vi "Set Line.vi"(8 "error in (no error)":errorcluster, 9 "Interlock Chain":refnum<class "Interlock Chain.lvclass">, 10 "Bit Field":u16, 11 "Storage Line in":refnum<class "Storage Line.lvclass">) -> (0 "error out":errorcluster, 3 "Storage Line out":refnum<class "Storage Line.lvclass">)   [LabVIEW 2015, in "cRIO-Carbondioxide.lvlib" / "CO2-Actor.lvlib" / "Storage Line.lvclass"]
uses:
  Storage Line.lvclass
  Interlocks/Interlock Chain/Interlock Chain.lvclass
  Storage Line.lvclass/Storage Line.ctl
  <vilib>/ActorFramework/Actor/Actor.lvclass/Actor.ctl
  <vilib>/ActorFramework/Message Enqueuer/Message Enqueuer.lvclass/Message Enqueuer.ctl
  Valve Messages/Write Bit Field Msg/Write Bit Field Msg.lvclass/Write Bit Field Msg.ctl
  <vilib>/ActorFramework/Actor/Read Self Enqueuer.vi
  <vilib>/ActorFramework/Message Enqueuer/Enqueue.vi
  Read Container.vi
  <vilib>/ActorFramework/Message Enqueuer/Init from Existing Queue.vi
  <vilib>/ActorFramework/Message Priority Queue/Priority Enqueue.vi
  Interlocks/Interlock/Interlock.lvclass
  <vilib>/ActorFramework/Actor/Actor.lvclass
  <vilib>/ActorFramework/Message Enqueuer/Message Enqueuer.lvclass
  Valve Messages/Write Bit Field Msg/Write Bit Field Msg.lvclass
  subs/Sample/Sample.lvclass
  CO2 Actor/CO2 Actor.lvclass
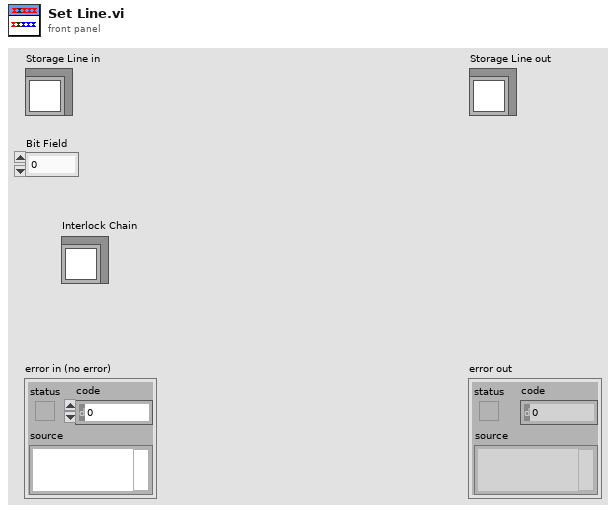
[diagram p1: front panel]
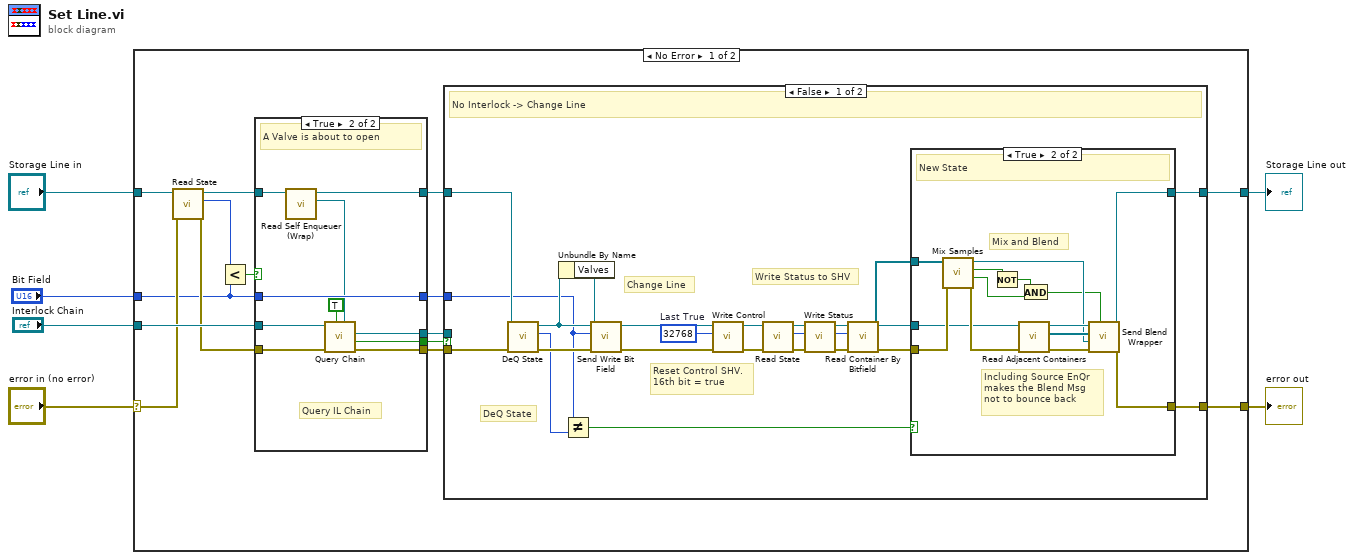
[diagram p0: block diagram]
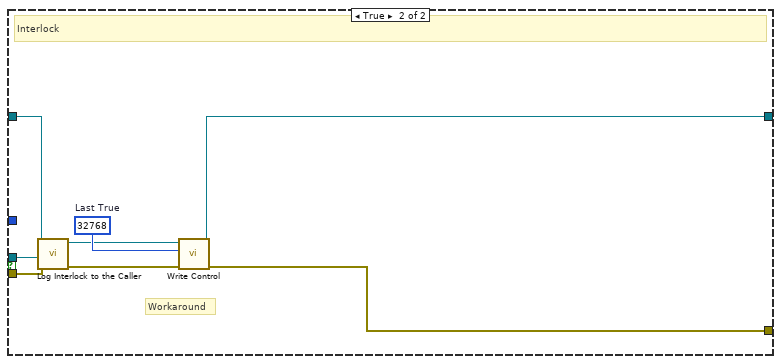
[diagram p4: hidden frame]
diagram:
  n1 = case shown="No Error" "error in (no error)" {
    selector: "error in (no error)" -> [w16 w83]
    tunnel: [w10 w83] -> w5
    tunnel: [w9 w82] -> w3
    tunnel: "Storage Line in" -> [w17 w82]
    tunnel: "Interlock Chain" -> [w21 _]
    tunnel: "Bit Field" -> [w13 _]
    frame No Error {
      n2 = call "Read State.vi"("error in (no error)"=w16, "Storage Line in"=w17) -> ("error out"=w15:errorcluster, "State"=w11:u16, "Storage Line out"=w8:refnum<class "Storage Line.lvclass">)  [unwired: 5 in, 2 out]
      n3 = Less?(x=w11, y=w13) -> (x < y?=w14:bool)
      n4 = case shown="True" w14 {
        tunnel: w21 -> [_ w34]
        tunnel: [w24 w32] -> w20
        tunnel: [_ w31] -> w19
        tunnel: [_ w30] -> w18
        tunnel: w15 -> [w24 w29]
        tunnel: w13 -> [w23 w28]
        tunnel: [w23 w28] -> w12
        tunnel: w8 -> [w22 w27]
        tunnel: [w22 w25] -> w7
        frame False {
          # "Nevermind Interlock"
          # "Valve is about to close"
        }
        frame True {
          # "Query IL Chain"
          # "A Valve is about to open"
          n5 = call "Read Self Enqueuer (Wrap).vi"("CO2 Actor in"=w27) -> ("Actor Framework:Message Enqueuer"=w26:refnum<class "Message Enqueuer.lvclass">, "CO2 Actor out"=w25:refnum<class "Storage Line.lvclass">)  [unwired: 9 in]
          n6 = call "Query Chain.vi"("Caller Enqueuer"=w26, "Close Connections (F)"=TRUE, "error in (no error)"=w29, "Interlock Chain"=w34) -> ("error out"=w32:errorcluster, "Interlock?"=w30:bool, "Interlock out"=w31:refnum<class "Interlock.lvclass">)  [unwired: 2 in, 3 out]
        }
      }
      n7 = case shown="False" w18 {
        tunnel: w12 -> [w37 _]
        tunnel: w7 -> [w43 w81]
        tunnel: [w55 w75] -> w9
        tunnel: w20 -> [w45 w80]
        tunnel: w19 -> [_ w79]
        tunnel: [w56 w74] -> w10
        frame False {
          w38 = u16 32768  # Last True
          # "Reset Control SHV.\n16th bit = true"
          # "DeQ State"
          # "Write Status to SHV"
          # "Change Line"
          # "No Interlock -> Change Line"
          n8 = call "DeQ State.vi"("error in (no error)"=w45, "Storage Line in"=w43) -> ("error out"=w44:errorcluster, "State"=w36:u16, "Storage Line out"=w40:refnum<class "Storage Line.lvclass">)  [unwired: 6 in, 1 out]
          n9 = Unbundle By Name(w40) -> ("Valves"=w57:refnum<class "Message Enqueuer.lvclass">)
          n10 = Not Equal?(x=w37, y=w36) -> (x != y?=w35:bool)
          n11 = call "Send Write Bit Field.vi"("error in (no error)"=w44, "Bit Field"=w37, "Message Enqueuer"=w57) -> ("error out"=w42:errorcluster)  [unwired: 5 in, 3 out]
          n12 = call "Write Control.vi"("error in (no error)"=w42, "Control"=w38, "Storage Line in"=w40) -> ("error out"=w41:errorcluster, "Storage Line out"=w39:refnum<class "Storage Line.lvclass">)  [unwired: 7 in]
          n13 = call "Read State.vi"("error in (no error)"=w41, "Storage Line in"=w39) -> ("error out"=w48:errorcluster, "State"=w47:u16, "Storage Line out"=w49:refnum<class "Storage Line.lvclass">)  [unwired: 5 in, 2 out]
          n14 = call "Write Status.vi"("error in (no error)"=w48, "Status Bitfield"=w47, "Storage Line in"=w49) -> ("error out"=w54:errorcluster, "Status Bitfield"=w46:u16, "Storage Line out"=w53:refnum<class "Storage Line.lvclass">)  [unwired: 6 in]
          n15 = call "Read Container By Bitfield.vi"("error in (no error)"=w54, "Bitfield"=w46, "Storage Line in"=w53) -> ("error out"=w52:errorcluster, "Samples"=w50:refnum<class "Sample.lvclass">[], "Storage Line out"=w51:refnum<class "Storage Line.lvclass">)  [unwired: 4 in, 2 out]
          n16 = case shown="True" w35 {
            tunnel: [w59 w68] -> w56
            tunnel: [w58 w67] -> w55
            tunnel: w52 -> [w59 w62]
            tunnel: w51 -> [w58 w61]
            tunnel: w50 -> [_ w60]
            frame False {
            }
            frame True {
              # "Including Source EnQr\nmakes the Blend Msg\nnot to bounce back"
              # "Mix and Blend"
              # "New State"
              n17 = call "Mix Samples.vi"("error in (no error)"=w62, "Samples In"=w60) -> ("error out"=w70:errorcluster, "is clean?"=w65:bool, "Empty Samples present?"=w64:bool, "Sample out"=w69:refnum<class "Sample.lvclass">)  [unwired: 6 in]
              n18 = Not(x=w64) -> (.not. x?=w63:bool)
              n19 = call "Read Adjacent Containers.vi"("error in (no error)"=w70, "Storage Line in"=w61) -> ("error out"=w73:errorcluster, "Adjacent Containers"=w71:refnum<class "Message Enqueuer.lvclass">[], "Storage Line out"=w72:refnum<class "Storage Line.lvclass">)  [unwired: 7 in]
              n20 = And(x=w63, y=w65) -> (x .and. y?=w66:bool)
              n21 = call-dynamic "Send Blend Wrapper.vi"("Include Source EnQr (T)"=w66, "error in (no error)"=w73, "Sample to Blend"=w69, "Send to"=w71, "CO2 Actor in"=w72) -> ("error out"=w68:errorcluster, "CO2 Actor out"=w67:refnum<class "Storage Line.lvclass">)  [unwired: 5 in]
            }
          }
        }
        frame True {
          w78 = u16 32768  # Last True
          # "Workaround"
          # "Interlock"
          n22 = call-dynamic "Log Interlock to the Caller.vi"("Interlock in"=w79, "error in (no error)"=w80, "CO2 Actor in"=w81) -> ("error out"=w77:errorcluster, "CO2 Actor out"=w76:refnum<class "Storage Line.lvclass">)  [unwired: 7 in]
          n23 = call "Write Control.vi"("error in (no error)"=w77, "Control"=w78, "Storage Line in"=w76) -> ("error out"=w74:errorcluster, "Storage Line out"=w75:refnum<class "Storage Line.lvclass">)  [unwired: 7 in]
        }
      }
    }
    frame Error {
    }
  }
  "error out" <- w5
  "Storage Line out" <- w3
